vi "main_pomiarowy.vi"() -> ()   [LabVIEW 2020]
uses:
  Kontrolki/Parametry_cosinusa.ctl
  Kontrolki/Parametry_cosinusow.ctl
  Kontrolki/Rodzaj_wzmacniacza.ctl
  Kontrolki/Dane.ctl
  Kontrolki/Rodzaj_modulacji.ctl
  <vilib>/measure/NI_MAPro.lvlib
  <vilib>/measure/maspectr.llb/FFT Spectrum (Mag-Phase) for 1 Chan.vi
  Kontrolki/Pasmo_przenoszenia.ctl
panel:
  in  "Pasmo_przenoszenia":T1
  out "Widmo_sygnalu_zdemodulowanego":cluster{"f0":dbl, "df":dbl, "magnitude":dbl[]}(graph)
  out "Moc_szczytowa":dbl
  out "Sprawnosc":dbl
  out "Moc_srednia":dbl
  out "Energia_sygnalu_zmodulowanego":waveform(dbl)(graph) caption="Waveform Chart 2"
  out "Moc_sygnalu_zmodulowanego":waveform(dbl)(graph) caption="Waveform Chart 2"
  out "Widmo_sygnalu_zmodulowanego":cluster{"f0":dbl, "df":dbl, "magnitude":dbl[]}[](graph)
  out "Sygnal_zmodulowany_i\nzmodulowany_rzeczywisty":waveform(dbl)[](graph) caption="Waveform Chart 2"
  out "Widmo_sygnalu_modulujacego":cluster{"f0":dbl, "df":dbl, "magnitude":dbl[]}(graph)
  out "Sygnal_modulujacy_i_zdemodulowany":waveform(dbl)[](graph) caption="Waveform Chart 2"
  in  "Rodzaj_modulacji":T2
  in  "Parametry_sygnalu_nosnego":T3={"Amplituda [V]"=1.0, "Czestotliwosc [Hz] "=2.0, "Faza [rad]"=0.0}
  in  "Rodzaj_wzmacniacza":T4
  in  "Wzmocnienie":dbl=1.0
  in  "Milisekund_na_dane":u32=20
  in  "stop":bool
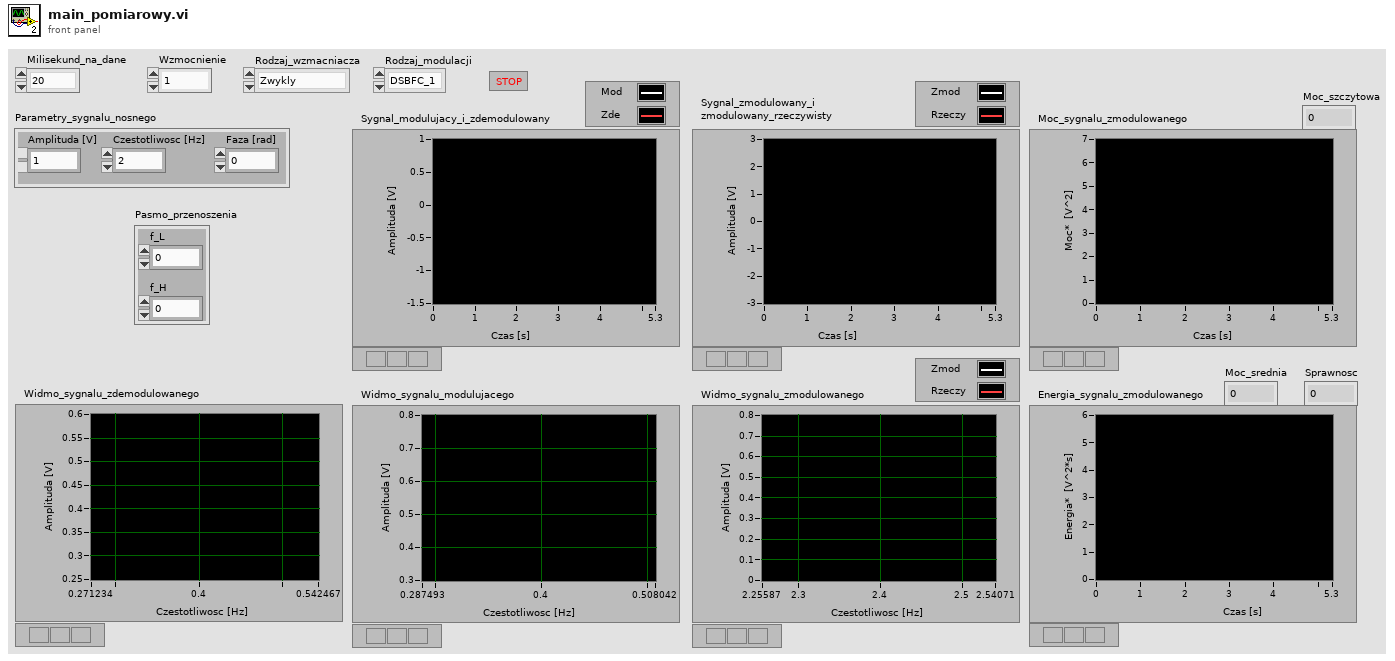
[diagram p1: front panel]
types:
  T1 = typedef "Pasmo_przenoszenia.ctl" = cluster{"f_L":dbl, "f_H":dbl}
  T2 = typedef "Rodzaj_modulacji.ctl" = enum16{"DSBFC_1", "DSBFC_2", "DSBSC", "USSBSC", "LSSBSC"}
  T3 = typedef "Parametry_cosinusa.ctl" = cluster{"Amplituda [V]":dbl, "Czestotliwosc [Hz] ":dbl, "Faza [rad]":dbl}
  T4 = typedef "Rodzaj_wzmacniacza.ctl" = enum16{"Zwykly", "Calkujacy", "Rozniczkujacy"}
  T5 = typedef "Dane.ctl" = cluster{"Parametry_sygnalu_modulujacego":T6, "Parametry_sygnalu_modulujacego_przesunietego":T6, "Sygnal_modulujacy_wzmocniony":dbl[], "Milisekund_na_dane":u32, "Wzmocnienie":dbl, "Rodzaj_wzmacniacza":T4, "Parametry_sygnalu_nosnego":T3, "Wektor_czasu":dbl[], "Sygnal_zmodulowany":dbl[], "Moc_sygnalu":dbl[], "Energia_sygnalu":dbl[], "Moc_szczytowa":dbl, "Sprawnosc":dbl, "Wartosc_poprzednia":dbl, "Czas":dbl, "Rodzaj_modulacji":T2, "Wartosc_poprzednia 2":dbl, "Moc_srednia":dbl, "Sygnal_zdemodulowany":dbl[], "Pasmo_przenoszenia":T1, "Rzeczywisty_sygnal":dbl[], "Rzeczywisty_zmodulowany":dbl[]}
  T6 = typedef "Parametry_cosinusow.ctl" = T3[]
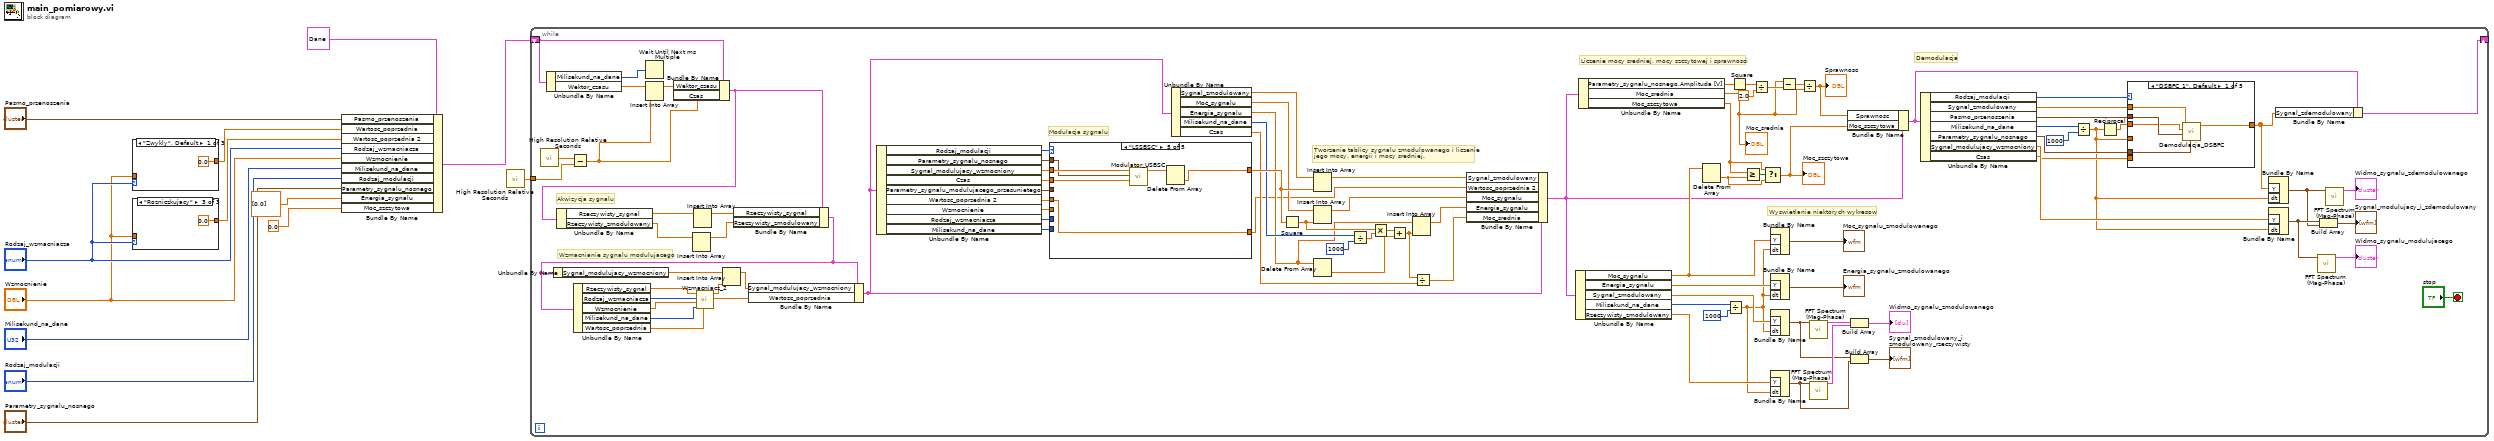
[diagram p0: block diagram]
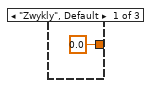
[diagram p2: hidden frame]
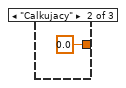
[diagram p3: hidden frame]
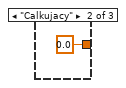
[diagram p4: hidden frame]
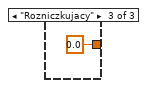
[diagram p5: hidden frame]
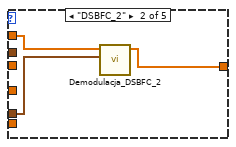
[diagram p6: hidden frame]
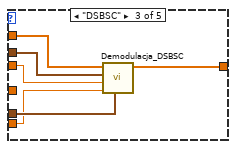
[diagram p7: hidden frame]
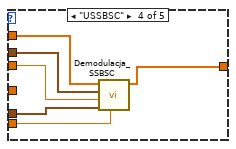
[diagram p8: hidden frame]
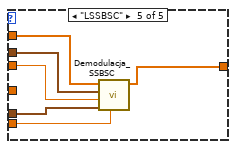
[diagram p9: hidden frame]
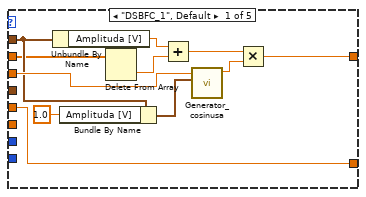
[diagram p10: hidden frame]
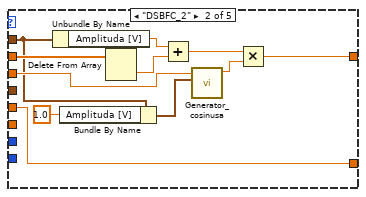
[diagram p11: hidden frame]
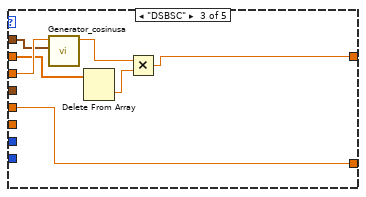
[diagram p12: hidden frame]
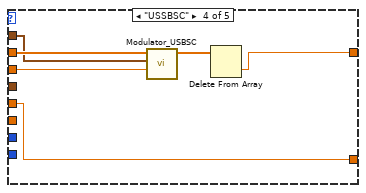
[diagram p13: hidden frame]
diagram:
  n1 = case shown="\"Zwykly\", Default" "Rodzaj_wzmacniacza" {
    tunnel: [0.0 ("Sygnal_modulujacy") 0.0 ("Sygnal_modulujacy") 0.0 ("Sygnal_modulujacy")] -> w7
    tunnel: "Wzmocnienie" -> [_ _ _]
    frame "Zwykly", Default {
    }
    frame "Calkujacy" {
    }
    frame "Rozniczkujacy" {
    }
  }
  n2 = case shown="\"Rozniczkujacy\"" "Rodzaj_wzmacniacza" {
    tunnel: [0.0 ("Sygnal_modulujacy") 0.0 ("Sygnal_modulujacy") 0.0 ("Sygnal_modulujacy")] -> w6
    tunnel: "Wzmocnienie" -> [_ _ _]
    frame "Zwykly", Default {
    }
    frame "Calkujacy" {
    }
    frame "Rozniczkujacy" {
    }
  }
  n3 = Bundle By Name(cluster=T5 {"Parametry_sygnalu_modulujacego"=[], "Parametry_sygnalu_modulujacego_przesunietego"=[], "Sygnal_modulujacy_wzmocniony"=[], "Milisekund_na_dane"=0, "Wzmocnienie"=0.0, "Rodzaj_wzmacniacza"=enum."Zwykly", "Parametry_sygnalu_nosnego"={"Amplituda [V]"=0.0, "Czestotliwosc [Hz] "=0.0, "Faza [rad]"=0.0}, "Wektor_czasu"=[], "Sygnal_zmodulowany"=[], "Moc_sygnalu"=[], "Energia_sygnalu"=[], "Moc_szczytowa"=0.0, "Sprawnosc"=0.0, "Wartosc_poprzednia"=0.0, "Czas"=0.0, "Rodzaj_modulacji"=enum."DSBFC_1", "Wartosc_poprzednia 2"=0.0, "Moc_srednia"=0.0, "Sygnal_zdemodulowany"=[], "Pasmo_przenoszenia"={"f_L"=0.0, "f_H"=0.0}, "Rzeczywisty_sygnal"=[], "Rzeczywisty_zmodulowany"=[]} ("Dane"), "Pasmo_przenoszenia"="Pasmo_przenoszenia", "Wartosc_poprzednia"=w7, "Wartosc_poprzednia 2"=w6, "Rodzaj_wzmacniacza"="Rodzaj_wzmacniacza", "Wzmocnienie"="Wzmocnienie", "Milisekund_na_dane"="Milisekund_na_dane", "Rodzaj_modulacji"="Rodzaj_modulacji", "Parametry_sygnalu_nosnego"="Parametry_sygnalu_nosnego", "Energia_sygnalu"=dbl[] [0.0], "Moc_szczytowa"=0.0) -> (w10:T5)
  n4 = call <vilib>:"High Resolution Relative Seconds.vi"() -> ("relative seconds"=w9:dbl)
  n5 = while {
    shift-right: [w42] -> _
    shift-left: w10 -> [w109]
    tunnel: w9 -> [w113]
    stop <- "stop" stop-if-true
    # "Akwizycja sygnalu"
    # "Wzmacnianie sygnalu modulujacego"
    # "Liczenie mocy sredniej, mocy szczytowej i sprawnosci"
    # "Wyswietlanie niektorych wykresow"
    # "Tworzenie tablicy sygnalu zmodulowanego i liczenie\njego mocy, energii i mocy sredniej."
    # "Demodulacja"
    # "Modulacja sygnalu"
    n6 = call <vilib>:"High Resolution Relative Seconds.vi"() -> ("relative seconds"=w114:dbl)
    n7 = Unbundle By Name(w109) -> ("Milisekund_na_dane"=w110:u32, "Wektor_czasu"=w112:dbl[])
    n8 = Subtract(x=w114, y=w113) -> (x-y=w20:dbl)
    n9 = Wait Until Next ms Multiple(millisecond multiple=w110) -> ()  [unwired: 1 out]
    n10 = Insert Into Array(array=w112, new element=w20) -> (w111:dbl[])  [unwired: 1 in]
    n11 = Bundle By Name(cluster=w109, "Wektor_czasu"=w111, "Czas"=w20) -> (w37:T5)
    n12 = Unbundle By Name(w37) -> ("Rzeczywisty_sygnal"=w39:dbl[], "Rzeczywisty_zmodulowany"=w38:dbl[])
    n13 = Insert Into Array(array=w38) -> (w35:dbl[])  [unwired: 2 in]
    n14 = Insert Into Array(array=w39) -> (w36:dbl[])  [unwired: 2 in]
    n15 = Bundle By Name(cluster=w37, "Rzeczywisty_sygnal"=w36, "Rzeczywisty_zmodulowany"=w35) -> (w29:T5)
    n16 = Unbundle By Name(w29) -> ("Sygnal_modulujacy_wzmocniony"=w100:dbl[])
    n17 = Unbundle By Name(w29) -> ("Rzeczywisty_sygnal"=w34:dbl[], "Rodzaj_wzmacniacza"=w33:T4, "Wzmocnienie"=w32:dbl, "Milisekund_na_dane"=w31:u32, "Wartosc_poprzednia"=w30:dbl)
    n18 = call "Wzmacniacz_2.vi"("Wartosc_poprzednia"=w30, "Milisekund_na_dane"=w31, "Wzmocnienie"=w32, "Rodzaj_wzmacniacza"=w33, "Sygnal_wejsciowy"=w34) -> ("Wartosc_poprzednia"=w94:dbl, "Sygnal_wzmocniony"=w93:dbl)  [unwired: 5 in]
    n19 = Insert Into Array(array=w100, new element=w93) -> (w99:dbl[])  [unwired: 1 in]
    n20 = Bundle By Name(cluster=w29, "Sygnal_modulujacy_wzmocniony"=w99, "Wartosc_poprzednia"=w94) -> (w98:T5)
    n21 = Unbundle By Name(w98) -> ("Rodzaj_modulacji"=w105:T2, "Parametry_sygnalu_nosnego"=w108:T3, "Sygnal_modulujacy_wzmocniony"=w97:dbl[], "Czas"=w107:dbl, "Parametry_sygnalu_modulujacego_przesunietego"=w106:T6, "Wartosc_poprzednia 2"=w104:dbl, "Wzmocnienie"=w103:dbl, "Rodzaj_wzmacniacza"=w102:T4, "Milisekund_na_dane"=w101:u32)
    n22 = case shown="\"LSSBSC\"" w105 {
      tunnel: w108 -> [w148 w155 w168 w173 w179]
      tunnel: w97 -> [w143 w158 w165 w174 w180]
      tunnel: w107 -> [w149 w156 w169 w172 w178]
      tunnel: [w141 w159 w164 w170 w176] -> w91
      tunnel: w106 -> [_ _ _ _ _]
      tunnel: w104 -> [w145 w152 w163 w175 w181]
      tunnel: w103 -> [_ _ _ _ _]
      tunnel: w102 -> [_ _ _ _ _]
      tunnel: w101 -> [_ _ _ _ _]
      tunnel: [w145 w152 w163 w175 w181] -> w66
      frame "DSBFC_1", Default {
        n23 = Unbundle By Name(w148) -> ("Amplituda [V]"=w151:dbl)
        n24 = Bundle By Name(cluster=w148, "Amplituda [V]"=1.0) -> (w146:T3)
        n25 = Delete From Array(array=w143) -> (deleted portion=w144:dbl)  [unwired: 2 in, 1 out]
        n26 = Add(x=w151, y=w144) -> (x+y=w142:dbl)
        n27 = call "Generator_cosinusa.vi"("Parametry_cosinusa"=w146, "Czas"=w149) -> ("A cos(2pift + phi)"=w150:dbl)  [unwired: 9 in]
        n28 = Multiply(x=w142, y=w150) -> (x*y=w141:dbl)
      }
      frame "DSBFC_2" {
        n29 = Unbundle By Name(w155) -> ("Amplituda [V]"=w162:dbl)
        n30 = Bundle By Name(cluster=w155, "Amplituda [V]"=1.0) -> (w153:T3)
        n31 = Delete From Array(array=w158) -> (deleted portion=w157:dbl)  [unwired: 2 in, 1 out]
        n32 = Add(x=w162, y=w157) -> (x+y=w161:dbl)
        n33 = call "Generator_cosinusa.vi"("Parametry_cosinusa"=w153, "Czas"=w156) -> ("A cos(2pift + phi)"=w160:dbl)  [unwired: 9 in]
        n34 = Multiply(x=w161, y=w160) -> (x*y=w159:dbl)
      }
      frame "DSBSC" {
        n35 = call "Generator_cosinusa.vi"("Parametry_cosinusa"=w168, "Czas"=w169) -> ("A cos(2pift + phi)"=w167:dbl)  [unwired: 9 in]
        n36 = Delete From Array(array=w165) -> (deleted portion=w166:dbl)  [unwired: 2 in, 1 out]
        n37 = Multiply(x=w167, y=w166) -> (x*y=w164:dbl)
      }
      frame "USSBSC" {
        n38 = call "Modulator_USBSC.vi"("Czas"=w172, "Parametry_sygnalu_nosnego"=w173, "Sygnal_modulujacy"=w174) -> ("Sygnal_zmodulowany"=w171:dbl[])  [unwired: 8 in]
        n39 = Delete From Array(array=w171) -> (deleted portion=w170:dbl)  [unwired: 2 in, 1 out]
      }
      frame "LSSBSC" {
        n40 = call "Modulator_USBSC.vi"("Czas"=w178, "Parametry_sygnalu_nosnego"=w179, "Sygnal_modulujacy"=w180) -> ("Sygnal_zmodulowany"=w177:dbl[])  [unwired: 8 in]
        n41 = Delete From Array(array=w177) -> (deleted portion=w176:dbl)  [unwired: 2 in, 1 out]
      }
    }
    n42 = Unbundle By Name(w98) -> ("Sygnal_zmodulowany"=w95:dbl[], "Moc_sygnalu"=w90:dbl[], "Energia_sygnalu"=w80:dbl[], "Milisekund_na_dane"=w84:u32, "Czas"=w77:dbl)
    n43 = Square(x=w91) -> (x^2=w86:dbl)
    n44 = Insert Into Array(array=w95, new element=w91) -> (w96:dbl[])  [unwired: 1 in]
    n45 = Insert Into Array(array=w90, new element=w86) -> (w89:dbl[])  [unwired: 1 in]
    n46 = Delete From Array(array=w80) -> (deleted portion=w81:dbl)  [unwired: 2 in, 1 out]
    n47 = Divide(x=w84, y=1000) -> (x/y=w83:dbl)
    n48 = Multiply(x=w86, y=w83) -> (x*y=w82:dbl)
    n49 = Add(x=w82, y=w81) -> (x+y=w76:dbl)
    n50 = Insert Into Array(array=w80, new element=w76) -> (w79:dbl[])  [unwired: 1 in]
    n51 = Divide(x=w76, y=w77) -> (x/y=w75:dbl)
    n52 = Bundle By Name(cluster=w98, "Sygnal_zmodulowany"=w96, "Wartosc_poprzednia 2"=w66, "Moc_sygnalu"=w89, "Energia_sygnalu"=w79, "Moc_srednia"=w75) -> (w41:T5)
    n53 = Unbundle By Name(w41) -> ("Moc_sygnalu"=w74:dbl[], "Energia_sygnalu"=w64:dbl[], "Sygnal_zmodulowany"=w43:dbl[], "Milisekund_na_dane"=w65:u32, "Rzeczywisty_zmodulowany"=w28:dbl[])
    n54 = Unbundle By Name(w41) -> ("Parametry_sygnalu_nosnego.Amplituda [V]"=w62:dbl, "Moc_srednia"=w57:dbl, "Moc_szczytowa"=w72:dbl)
    "Moc_srednia" <- w57
    n55 = Delete From Array(array=w74) -> (deleted portion=w63:dbl)  [unwired: 2 in, 1 out]
    n56 = Divide(x=w65, y=1000) -> (x/y=w27:dbl)
    n57 = Square(x=w62) -> (x^2=w61:dbl)
    n58 = Greater Or Equal?(x=w72, y=w63) -> (x >= y?=w73:bool)
    n59 = Divide(x=w61, y=2.0) -> (x/y=w59:dbl)
    n60 = Select(t=w72, s=w73, f=w63) -> (s? t:f=w71:dbl)
    "Moc_szczytowa" <- w71
    n61 = Bundle By Name("Y"=w74, "dt"=w27) -> (→"Moc_sygnalu_zmodulowanego":waveform(dbl))  [unwired: 1 in]
    n62 = Bundle By Name("Y"=w64, "dt"=w27) -> (→"Energia_sygnalu_zmodulowanego":waveform(dbl))  [unwired: 1 in]
    n63 = Bundle By Name("Y"=w43, "dt"=w27) -> (w22:waveform(dbl))  [unwired: 1 in]
    n64 = Bundle By Name("Y"=w28, "dt"=w27) -> (w21:waveform(dbl))  [unwired: 1 in]
    n65 = Subtract(x=w57, y=w59) -> (x-y=w58:dbl)
    n66 = Divide(x=w58, y=w57) -> (x/y=w54:dbl)
    "Sprawnosc" <- w54
    n67 = call-poly <vilib>:"FFT Spectrum (Mag-Phase).vi"("time signal"=w22) -> ("magnitude"=w23:cluster{"f0":dbl, "df":dbl, "magnitude":dbl[]})  [unwired: 6 in, 4 out]
    n68 = call-poly <vilib>:"FFT Spectrum (Mag-Phase).vi"("time signal"=w21) -> ("magnitude"=w24:cluster{"f0":dbl, "df":dbl, "magnitude":dbl[]})  [unwired: 6 in, 4 out]
    n69 = Bundle By Name(cluster=w41, "Sprawnosc"=w54, "Moc_szczytowa"=w71) -> (w67:T5)
    n70 = Build Array(w23, w24) -> (→"Widmo_sygnalu_zmodulowanego":cluster{"f0":dbl, "df":dbl, "magnitude":dbl[]}[])
    n71 = Build Array(w22, w21) -> (→"Sygnal_zmodulowany_i\nzmodulowany_rzeczywisty":waveform(dbl)[])
    n72 = Unbundle By Name(w67) -> ("Rodzaj_modulacji"=w48:T2, "Sygnal_zmodulowany"=w52:dbl[], "Pasmo_przenoszenia"=w51:T1, "Milisekund_na_dane"=w69:u32, "Parametry_sygnalu_nosnego"=w49:T3, "Sygnal_modulujacy_wzmocniony"=w50:dbl[], "Czas"=w46:dbl)
    n73 = Divide(x=w69, y=u32 1000) -> (x/y=w40:dbl)
    n74 = Reciprocal(x=w40) -> (1/x=w47:dbl)
    n75 = case shown="\"DSBFC_1\", Default" w48 {
      tunnel: w52 -> [w119 w121 w124 w134 w140]
      tunnel: w51 -> [w118 _ w126 w133 w139]
      tunnel: w49 -> [w117 w122 w128 w130 w136]
      tunnel: [w116 w120 w123 w132 w138] -> w45
      tunnel: w47 -> [w115 _ w125 w131 w137]
      tunnel: w40 -> [_ _ _ _ _]
      tunnel: w46 -> [_ _ w127 w129 w135]
      frame "DSBFC_1", Default {
        n76 = call "Demodulacja_DSBFC.vi"("Parametry_sygnalu_nosnego"=w117, "Pasmo_przenoszenia"=w118, "Czestotliwosc_probkowania"=w115, "Sygnal_zmodulowany"=w119) -> ("Sygnal_zdemodulowany"=w116:dbl[])  [unwired: 7 in]
      }
      frame "DSBFC_2" {
        n77 = call "Demodulacja_DSBFC_2.vi"("Parametry_sygnalu_nosnego"=w122, "Sygnal_zmodulowany"=w121) -> ("Sygnal_zdemodulowany"=w120:dbl[])  [unwired: 9 in]
      }
      frame "DSBSC" {
        n78 = call "Demodulacja_DSBSC.vi"("Sygnal_zmodulowany"=w124, "Pasmo_przenoszenia"=w126, "Czestotliwosc_probkowania"=w125, "Czas"=w127, "Parametry_sygnalu_nosnego"=w128) -> ("Sygnal_zdemodulowany"=w123:dbl[])  [unwired: 5 in]
      }
      frame "USSBSC" {
        n79 = call "Demodulacja_SSBSC.vi"("Czas"=w129, "Parametry_sygnalu_nosnego"=w130, "Czestotliwosc_probkowania"=w131, "Pasmo_przenoszenia"=w133, "Sygnal_zmodulowany"=w134) -> ("Sygnal_zdemodulowany"=w132:dbl[])  [unwired: 6 in]
      }
      frame "LSSBSC" {
        n80 = call "Demodulacja_SSBSC.vi"("Czas"=w135, "Parametry_sygnalu_nosnego"=w136, "Czestotliwosc_probkowania"=w137, "Pasmo_przenoszenia"=w139, "Sygnal_zmodulowany"=w140) -> ("Sygnal_zdemodulowany"=w138:dbl[])  [unwired: 6 in]
      }
    }
    n81 = Bundle By Name("Y"=w45, "dt"=w40) -> (w44:waveform(dbl))  [unwired: 1 in]
    n82 = Bundle By Name("Y"=w50, "dt"=w40) -> (w56:waveform(dbl))  [unwired: 1 in]
    n83 = Bundle By Name(cluster=w67, "Sygnal_zdemodulowany"=w45) -> (w42:T5)
    n84 = call-poly <vilib>:"FFT Spectrum (Mag-Phase).vi"("time signal"=w56) -> ("magnitude"=→"Widmo_sygnalu_modulujacego":cluster{"f0":dbl, "df":dbl, "magnitude":dbl[]})  [unwired: 6 in, 4 out]
    n85 = Build Array(w56, w44) -> (→"Sygnal_modulujacy_i_zdemodulowany":waveform(dbl)[])
    n86 = call-poly <vilib>:"FFT Spectrum (Mag-Phase).vi"("time signal"=w44) -> ("magnitude"=→"Widmo_sygnalu_zdemodulowanego":cluster{"f0":dbl, "df":dbl, "magnitude":dbl[]})  [unwired: 6 in, 4 out]
  }
